vi "Dynamic VI.vi"() -> ()   [LabVIEW 2012]
panel:
  out "Accelerometer Graph":dynamicdata(graph)
  in  "Save To File:":path=path "C:/scratch/JT/MEL3/Lab2Data.lvm" caption="Filename"
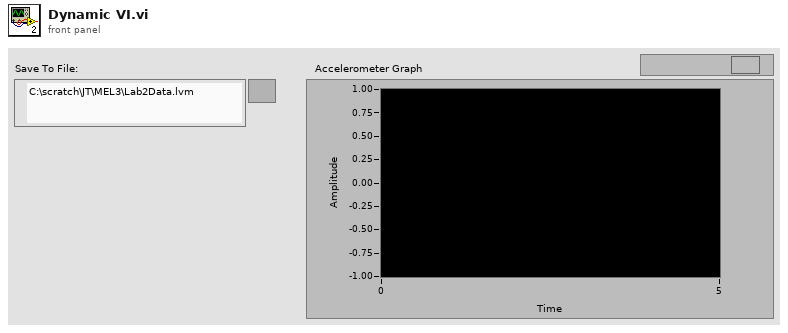
[diagram p1: front panel]
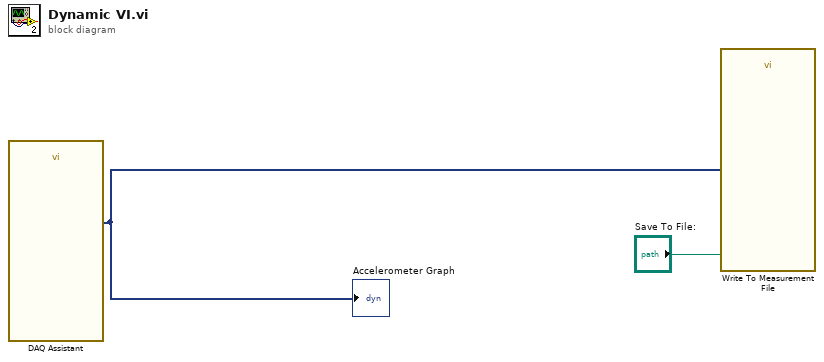
[diagram p0: block diagram]
diagram:
  n1 = call "DAQ Assistant"() -> ("data"=w1:dynamicdata)  [unwired: 17 in, 2 out]
  "Accelerometer Graph" <- w1
  n2 = call "Write To Measurement File"("Signals"=w1, "Filename"="Save To File:") -> ()  [unwired: 15 in, 3 out]
